vi "Array to Signal.vi"(0 "I2C in":refnum<class "I2C.lvclass">, 5 "Data Array":bool[](array[boolean]), 11 "Error In":errorcluster) -> (4 "I2C out":refnum<class "I2C.lvclass">, 15 "Error Out":errorcluster)   [LabVIEW 2020, in "I2C Controller.lvlib" / "I2C.lvclass"]
doc: "This Subvi is used to write the array of boolean data into the waveform data and the transitions"
uses:
  I2C.lvclass
  I2C.lvclass/I2C.ctl
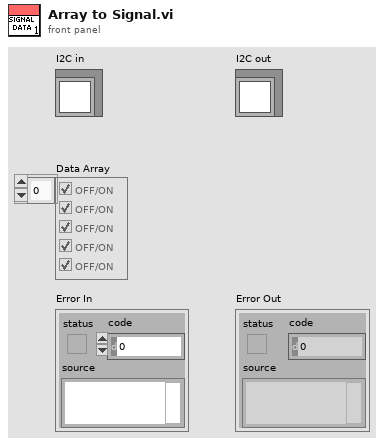
[diagram p1: front panel]
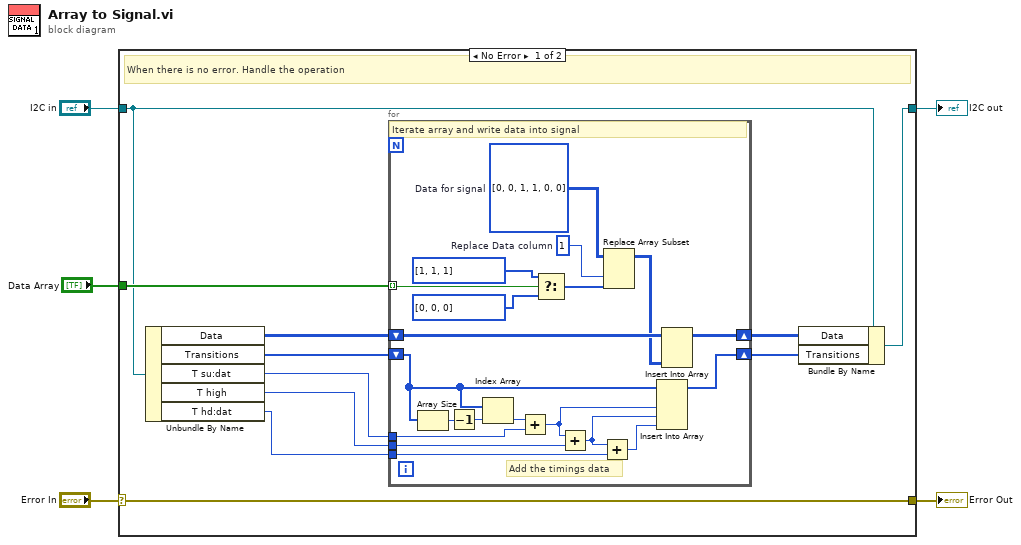
[diagram p0: block diagram]
diagram:
  n1 = case shown="No Error" "Error In" {
    selector: "Error In" -> [w16 w38]
    tunnel: [w16 w38] -> w4
    tunnel: [w8 w37] -> w2
    tunnel: "I2C in" -> [w9 w37]
    tunnel: "Data Array" -> [w10 _]
    frame No Error {
      # "When there is no error. Handle the operation"
      n2 = Unbundle By Name(w9) -> ("Data"=w15:u8[][], "Transitions"=w14:u32[], "T su:dat"=w13:u32, "T high"=w12:u32, "T hd:dat"=w11:u32)
      n3 = for {
        shift-right: [w34] -> w7
        shift-left: w15 -> [w36]
        shift-right: [w35] -> w6
        shift-left: w14 -> [w33]
        tunnel: w13 -> [w29]
        tunnel: w12 -> [w28]
        tunnel: w11 -> [w25]
        tunnel: w10 -> [w23] mode=indexing
        w19 = 1  # Replace Data column
        w20 = u8[][] [[0, 0], [1, 1], [0, 0]]  # Data for signal
        # "Add the timings data"
        # "Iterate array and write data into signal"
        n4 = Array Size(array=w33) -> (size(s)=w32:i32)
        n5 = Decrement(x=w32) -> (x-1=w31:i32)
        n6 = Index Array(array=w33, index=w31) -> (element=w30:u32)
        n7 = Add(x=w30, y=w29) -> (x+y=w27:u32)
        n8 = Select(t=u8[] [1, 1, 1] ("Data"), s=w23, f=u8[] [0, 0, 0] ("Data")) -> (s? t:f=w18:u8[])
        n9 = Add(x=w27, y=w28) -> (x+y=w26:u32)
        n10 = Add(x=w26, y=w25) -> (x+y=w24:u32)
        n11 = Replace Array Subset(array=w20, new element=w18, index (col)=w19) -> (w17:u8[][])  [unwired: 1 in]
        n12 = Insert Into Array(array=w33, new element #1=w27, new element #2=w26, new element #3=w24) -> (w35:u32[])  [unwired: 1 in]
        n13 = Insert Into Array(array=w36, new element=w17) -> (w34:u8[][])  [unwired: 2 in]
      }
      n14 = Bundle By Name(cluster=w9, "Data"=w7, "Transitions"=w6) -> (w8:refnum<class "I2C.lvclass">)
    }
    frame Error {
      # "when there is error. do nothing."
    }
  }
  "Error Out" <- w4
  "I2C out" <- w2
